vi "20151117 Action limiter.vi"(4 "Actions":i16[](array[numeric])) -> (1 "Action limiter":T1)   [LabVIEW 2013]
panel:
  # "When upper limit reached the actions can take"
  # "When lower limit reached the actions can take"
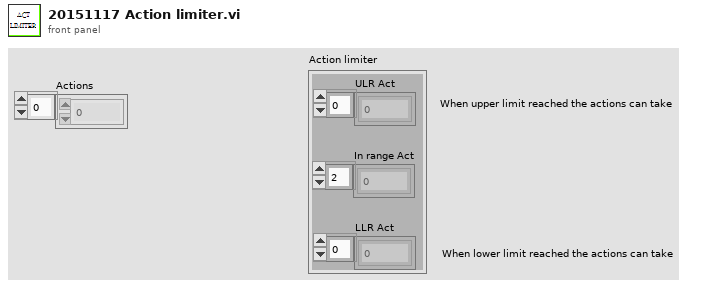
[diagram p1: front panel]
types:
  T1 = cluster{"LLR Act":i16[], "ULR Act":i16[], "In range Act":i16[]}
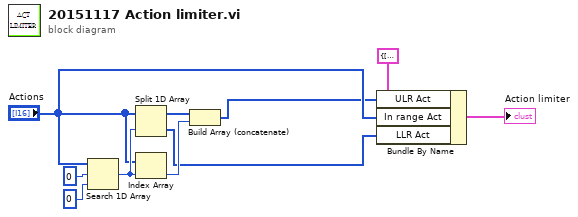
[diagram p0: block diagram]
diagram:
  n1 = Search 1D Array(1D array="Actions", element=i16 0, start index (0)=0) -> (index of element=w8:i32)
  n2 = Split 1D Array(array="Actions", index=w8) -> (first subarray=w6:i16[], second subarray=w3:i16[])
  n3 = Index Array(array="Actions", index=w8) -> (element=w7:i16)
  n4 = Build Array (concatenate)(w6, w7) -> (w2:i16[])
  n5 = Bundle By Name(cluster=T1 {"LLR Act"=[0], "ULR Act"=[], "In range Act"=[]} ("Cluster"), "ULR Act"=w2, "In range Act"="Actions", "LLR Act"=w3) -> (→"Action limiter":T1)
